vi "sensors.vi"() -> ()   [LabVIEW 2019]
panel:
  out "Setpoint Shooter":dbl
  out "Wheel_4 (deg)":dbl
  out "Wheel_3 (deg)":dbl
  out "Wheel_2 (deg)":dbl
  out "Wheel_1 (deg)":dbl
  out "Robot_H (deg)":dbl
  out "Set_Robot_H (deg)":dbl
  out "Set_Robot_Pos":bool
  out "Set_Robot_Y (in)":dbl
  out "Set_Robot_X (in)":dbl
  out "Distance_From_Start (in)":dbl
  out "Robot_Y (in)":dbl
  out "Robot_X (in)":dbl
  out "EncoderVel_Right_Drive (ft/sec)":dbl
  out "EncoderVel_Left_Drive (ft/sec)":dbl
  out "Absolute_Distance (in)":dbl
  out "Distance_From_End (in)":dbl
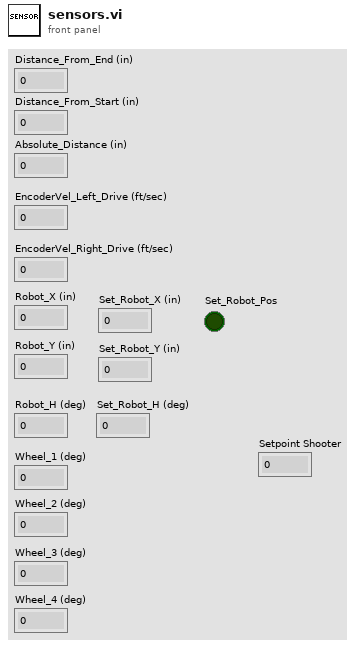
[diagram p1: front panel]
diagram:
